vi "Rollers Logic Test.vi"() -> ()   [LabVIEW 2013]
uses:
  Robot Code/Rollers/Roller Control.ctl
  Robot Code/Rollers/Roller Mode.ctl
  <vilib>/Rock Robotics/WPI/Solenoid/WPI_SolenoidValue.ctl
panel:
  out "Back Solenoid":T1
  out "Back Motor":dbl
  out "Front Solenoid":T1
  out "Front Motor":dbl
  in  "Roller Command":T2
  in  "stop":bool
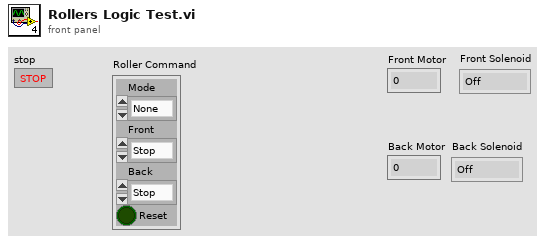
[diagram p1: front panel]
types:
  T1 = typedef "WPI_SolenoidValue.ctl" = enum16{"Off", "On", "Forward", "Reverse"}
  T2 = typedef "Roller Control.ctl" = cluster{"Mode":T3, "Front":enum16{"Stop", "Forward", "Reverse"}, "Back":enum16{"Stop", "Forward", "Reverse"}, "Reset":bool}
  T3 = typedef "Roller Mode.ctl" = enum16{"None", "Front", "Back", "Both", "Manual"}
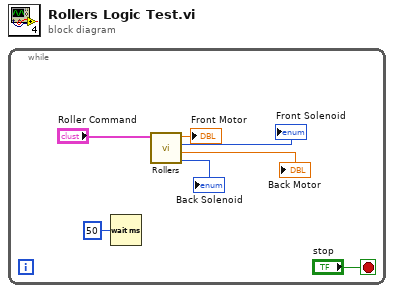
[diagram p0: block diagram]
diagram:
  n1 = while {
    stop <- "stop" stop-if-true
    n2 = Wait (ms)(milliseconds to wait=u32 50) -> ()  [unwired: 1 out]
    n3 = call "Rollers.vi"("Roller Command"="Roller Command") -> ("Back Solenoid"=→"Back Solenoid":T1, "Back Motor"=→"Back Motor":dbl, "Front Solenoid"=→"Front Solenoid":T1, "Front Motor"=→"Front Motor":dbl)  [unwired: 7 in]
  }
